vi "enter_array.vi"(0 "future?":bool=TRUE, 3 "Cursor IN":i32[](array[numeric]), 4 "ItemNames in":string[][](array[string]), 5 "array":string[][](array[string])) -> (1 "Cursor OUT":i32[](array[numeric]), 2 "ItemNames out":string[][](array[string]))   [LabVIEW 2020]
panel:
  # "About This VI:\nWhen \"future event?\" is ON,  this VI does the followings.\n- First read \"ItemNames in\" then add \"Array\" which has the same column dimension\n- In parallel,  read \"Value\" which is the position of the highlighted cursor in upper VI then +1 and produce \"val(sgnl)\"\n* \"Value\" and \"val(sgnl)\" are in 1D array, however we only concern the  0th value. \n\nWhen \"future event?\" is OFF, send the message  'You cannot edit the current or past sequence.'"
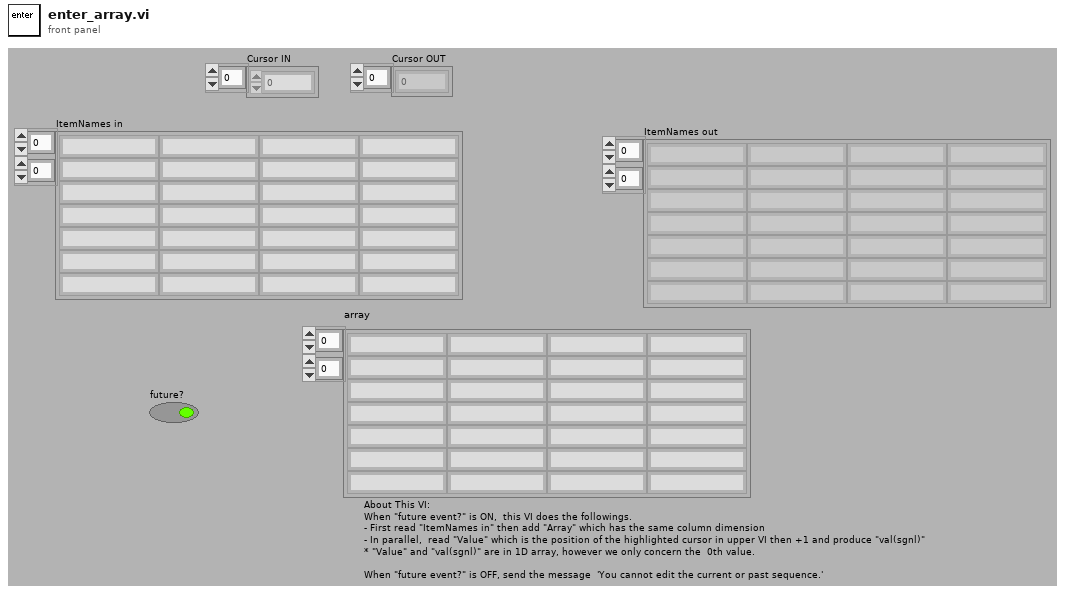
[diagram p1: front panel]
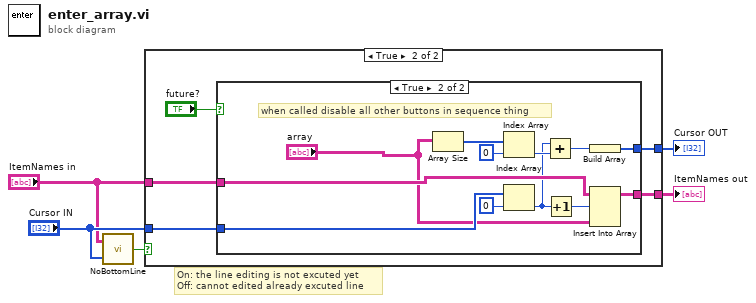
[diagram p0: block diagram]
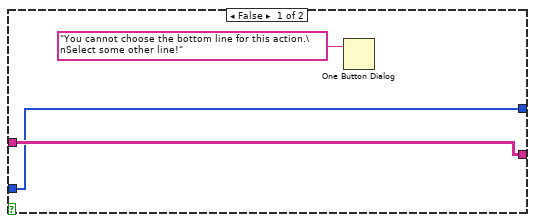
[diagram p2: hidden frame]
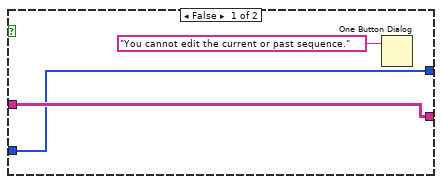
[diagram p3: hidden frame]
diagram:
  # "On: the line editing is not excuted yet\nOff: cannot edited already excuted line"
  n1 = call "NoBottomLine.vi"("Value in"="Cursor IN", "ItemNames in"="ItemNames in") -> ("no bottom?"=w2:bool)
  n2 = case shown="True" w2 {
    tunnel: "ItemNames in" -> [w8 w13]
    tunnel: "Cursor IN" -> [w7 w12]
    tunnel: [w8 w11] -> w5
    tunnel: [w7 w9] -> w1
    frame False {
      n3 = One Button Dialog(message="You cannot choose the bottom line for this action.\nSelect some other line!") -> ()  [unwired: 1 in, 1 out]
    }
    frame True {
      n4 = case shown="True" "future?" {
        tunnel: w13 -> [w16 w28]
        tunnel: [w16 w27] -> w11
        tunnel: w12 -> [w14 w26]
        tunnel: [w14 w25] -> w9
        frame False {
          n5 = One Button Dialog(message="You cannot edit the current or past sequence.") -> ()  [unwired: 1 in, 1 out]
        }
        frame True {
          # "when called disable all other buttons in sequence thing"
          n6 = Array Size(array="array") -> (size(s)=w22:i32[])
          n7 = Index Array(array=w22, index=0) -> (element=w20:i32)
          n8 = Index Array(array=w26, index=0) -> (element=w18:i32)
          n9 = Add(x=w18, y=w20) -> (x+y=w21:i32)
          n10 = Increment(x=w18) -> (x+1=w19:i32)
          n11 = Build Array(w21) -> (w25:i32[])
          n12 = Insert Into Array(array=w28, index (row)=w19, new element="array") -> (w27:string[][])  [unwired: 1 in]
        }
      }
    }
  }
  "ItemNames out" <- w5
  "Cursor OUT" <- w1
